vi "Battleship_Init.vi"(0 "object in":refnum<class "Battleship.lvclass">, 2 "ShipType":T2, 3 "GameType":T1, 5 "error in (no error)":errorcluster) -> (14 "object out":refnum<class "Battleship.lvclass">, 19 "error out":errorcluster)   [LabVIEW 2015, in "Battleship.lvclass"]
uses:
  Battleship.lvclass
  TypDefs/ShipType.ctl
  TypDefs/GameType.ctl
  TypDefs/Coordinates.ctl
  Battleship.lvclass/Battleship.ctl
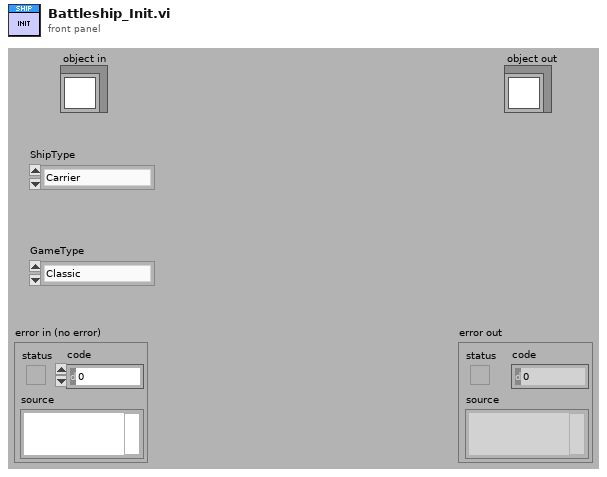
[diagram p1: front panel]
types:
  T1 = typedef "GameType.ctl" = enum16{"Classic", "Modern"}
  T2 = typedef "ShipType.ctl" = enum16{"Carrier", "Destroyer", "Submarine", "Frigate", "Scout"}
  T3 = typedef "Coordinates.ctl" = cluster{"X":i32, "Y":i32}
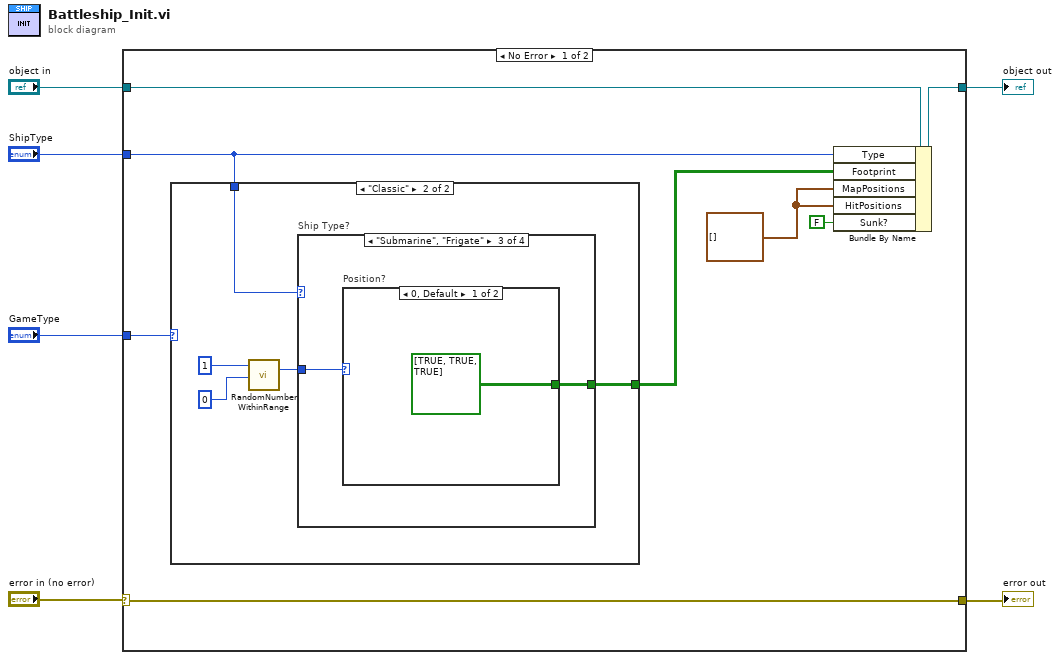
[diagram p0: block diagram]
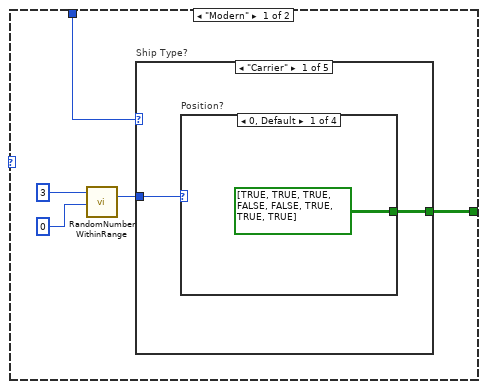
[diagram p2: hidden frame]
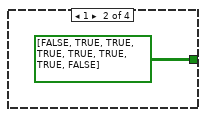
[diagram p3: hidden frame]
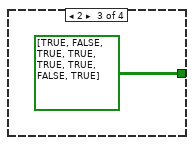
[diagram p4: hidden frame]
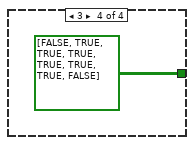
[diagram p5: hidden frame]
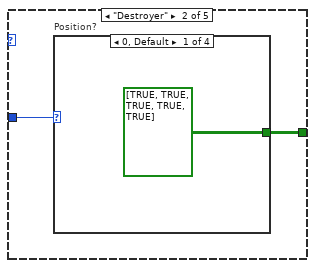
[diagram p6: hidden frame]
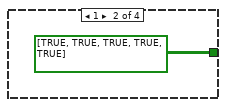
[diagram p7: hidden frame]
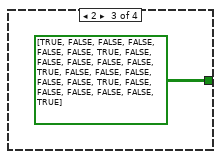
[diagram p8: hidden frame]
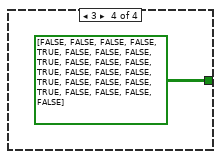
[diagram p9: hidden frame]
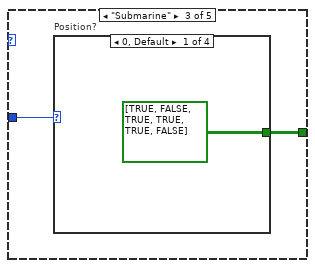
[diagram p10: hidden frame]
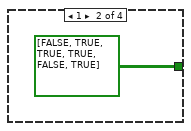
[diagram p11: hidden frame]
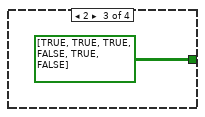
[diagram p12: hidden frame]
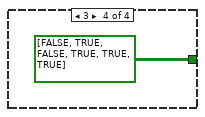
[diagram p13: hidden frame]
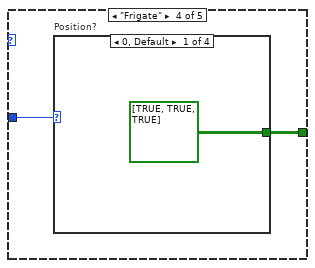
[diagram p14: hidden frame]
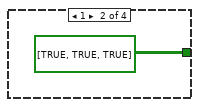
[diagram p15: hidden frame]
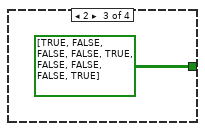
[diagram p16: hidden frame]
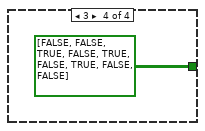
[diagram p17: hidden frame]
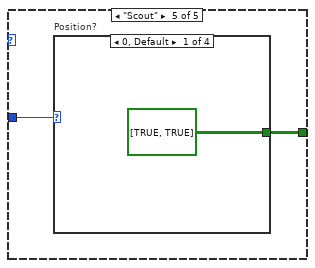
[diagram p18: hidden frame]
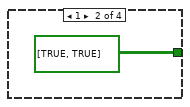
[diagram p19: hidden frame]
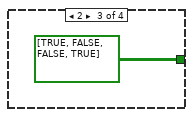
[diagram p20: hidden frame]
diagram:
  n1 = case shown="No Error" "error in (no error)" {
    selector: "error in (no error)" -> [w12 w71]
    tunnel: "object in" -> [w14 w72]
    tunnel: [w13 w72] -> w5
    tunnel: [w12 w71] -> w3
    tunnel: "ShipType" -> [w11 _]
    tunnel: "GameType" -> [w7 _]
    frame No Error {
      w9 = T3[] [] ("MapPositions")
      n2 = case shown="\"Classic\"" w7 {
        tunnel: w11 -> [w19 w54]
        tunnel: [w18 w53] -> w10
        frame "Modern" {
          n3 = call "RandomNumberWithinRange.vi"("High"=3, "Low"=0) -> ("Random Number"=w17:i32)  [unwired: 25 in]
          n4 = case "Ship Type?" shown="\"Carrier\"" w19 {
            tunnel: [w21 w27 w33 w39 w45] -> w18
            tunnel: w17 -> [w20 w26 w32 w38 w44]
            frame "Carrier" {
              n5 = case "Position?" shown="0, Default" w20 {
                tunnel: [bool[][] [[TRUE, TRUE, TRUE, FALSE], [FALSE, TRUE, TRUE, TRUE]] bool[][] [[FALSE, TRUE, TRUE, TRUE], [TRUE, TRUE, TRUE, FALSE]] bool[][] [[TRUE, FALSE], [TRUE, TRUE], [TRUE, TRUE], [FALSE, TRUE]] bool[][] [[FALSE, TRUE], [TRUE, TRUE], [TRUE, TRUE], [TRUE, FALSE]]] -> w21
                frame 0, Default {
                }
                frame 1 {
                }
                frame 2 {
                }
                frame 3 {
                }
              }
            }
            frame "Destroyer" {
              n6 = case "Position?" shown="0, Default" w26 {
                tunnel: [bool[][] [[TRUE], [TRUE], [TRUE], [TRUE], [TRUE]] bool[][] [[TRUE, TRUE, TRUE, TRUE, TRUE]] bool[][] [[TRUE, FALSE, FALSE, FALSE, FALSE], [FALSE, TRUE, FALSE, FALSE, FALSE], [FALSE, FALSE, TRUE, FALSE, FALSE], [FALSE, FALSE, FALSE, TRUE, FALSE], [FALSE, FALSE, FALSE, FALSE, TRUE]] bool[][] [[FALSE, FALSE, FALSE, FALSE, TRUE], [FALSE, FALSE, FALSE, TRUE, FALSE], [FALSE, FALSE, TRUE, FALSE, FALSE], [FALSE, TRUE, FALSE, FALSE, FALSE], [TRUE, FALSE, FALSE, FALSE, FALSE]]] -> w27
                frame 0, Default {
                }
                frame 1 {
                }
                frame 2 {
                }
                frame 3 {
                }
              }
            }
            frame "Submarine" {
              n7 = case "Position?" shown="0, Default" w32 {
                tunnel: [bool[][] [[TRUE, FALSE], [TRUE, TRUE], [TRUE, FALSE]] bool[][] [[FALSE, TRUE], [TRUE, TRUE], [FALSE, TRUE]] bool[][] [[TRUE, TRUE, TRUE], [FALSE, TRUE, FALSE]] bool[][] [[FALSE, TRUE, FALSE], [TRUE, TRUE, TRUE]]] -> w33
                frame 0, Default {
                }
                frame 1 {
                }
                frame 2 {
                }
                frame 3 {
                }
              }
            }
            frame "Frigate" {
              n8 = case "Position?" shown="0, Default" w38 {
                tunnel: [bool[][] [[TRUE], [TRUE], [TRUE]] bool[][] [[TRUE, TRUE, TRUE]] bool[][] [[TRUE, FALSE, FALSE], [FALSE, TRUE, FALSE], [FALSE, FALSE, TRUE]] bool[][] [[FALSE, FALSE, TRUE], [FALSE, TRUE, FALSE], [TRUE, FALSE, FALSE]]] -> w39
                frame 0, Default {
                }
                frame 1 {
                }
                frame 2 {
                }
                frame 3 {
                }
              }
            }
            frame "Scout" {
              n9 = case "Position?" shown="0, Default" w44 {
                tunnel: [bool[][] [[TRUE], [TRUE]] bool[][] [[TRUE, TRUE]] bool[][] [[TRUE, FALSE], [FALSE, TRUE]] bool[][] [[FALSE, TRUE], [TRUE, FALSE]]] -> w45
                frame 0, Default {
                }
                frame 1 {
                }
                frame 2 {
                }
                frame 3 {
                }
              }
            }
          }
        }
        frame "Classic" {
          n10 = call "RandomNumberWithinRange.vi"("High"=1, "Low"=0) -> ("Random Number"=w52:i32)  [unwired: 25 in]
          n11 = case "Ship Type?" shown="\"Submarine\", \"Frigate\"" w54 {
            tunnel: [w56 w60 w64 w68] -> w53
            tunnel: w52 -> [w55 w59 w63 w67]
            frame "Carrier" {
              n12 = case "Position?" shown="1" w55 {
                tunnel: [bool[][] [[TRUE, TRUE, TRUE, TRUE, TRUE]] bool[][] [[TRUE], [TRUE], [TRUE], [TRUE], [TRUE]]] -> w56
                frame 0, Default {
                }
                frame 1 {
                }
              }
            }
            frame "Destroyer" {
              n13 = case "Position?" shown="0, Default" w59 {
                tunnel: [bool[][] [[TRUE], [TRUE], [TRUE], [TRUE]] bool[][] [[TRUE, TRUE, TRUE, TRUE]]] -> w60
                frame 0, Default {
                }
                frame 1 {
                }
              }
            }
            frame "Submarine", "Frigate" {
              n14 = case "Position?" shown="0, Default" w63 {
                tunnel: [bool[][] [[TRUE], [TRUE], [TRUE]] bool[][] [[TRUE, TRUE, TRUE]]] -> w64
                frame 0, Default {
                }
                frame 1 {
                }
              }
            }
            frame "Scout" {
              n15 = case "Position?" shown="0, Default" w67 {
                tunnel: [bool[][] [[TRUE], [TRUE]] bool[][] [[TRUE, TRUE]]] -> w68
                frame 0, Default {
                }
                frame 1 {
                }
              }
            }
          }
        }
      }
      n16 = Bundle By Name(cluster=w14, "Type"=w11, "Footprint"=w10, "MapPositions"=w9, "HitPositions"=w9, "Sunk?"=FALSE) -> (w13:refnum<class "Battleship.lvclass">)
    }
    frame Error {
    }
  }
  "object out" <- w5
  "error out" <- w3
